vi "Write Input Action.vi"(8 "Error In":errorcluster, 10 "Input Action":T1, 11 "XBMC Ref":T2) -> (0 "Error Out":errorcluster, 3 "XBMC Ref":T2)   [LabVIEW 2013, in "LVH-XBMC.lvlib"]
uses:
  <vilib>/LabVIEW Hacker/XBMC/LVH-XBMC.lvlib
  <vilib>/LabVIEW Hacker/XBMC/Private/Type Defs/XBMC Ref.ctl
  <vilib>/httpClient/ClientHandle.ctl
  <vilib>/LabVIEW Hacker/XBMC/Private/Type Defs/Input.Action.ctl
  <vilib>/httpClient/LabVIEWHTTPClient.lvlib
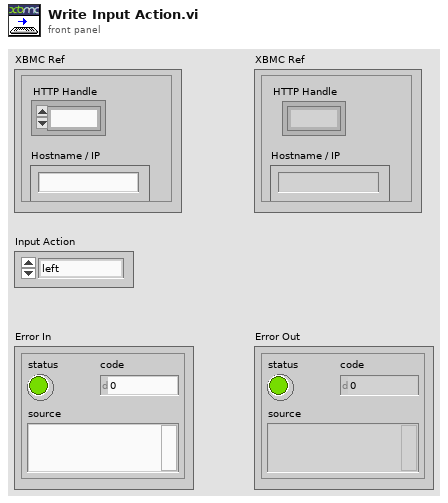
[diagram p1: front panel]
types:
  T1 = typedef "LVH-XBMC.lvlib/Input.Action.ctl" = enum16{"left", "right", "up", "down", "pageup", "pagedown", "select", "highlight", "parentdir", "parentfolder", "back", "previousmenu", "info", "pause", "stop", "skipnext", "skipprevious", "fullscreen", "aspectratio", "stepforward", "stepback", "bigstepforward", "bigstepback", "chapterorbigstepforward", "chapterorbigstepback", "osd", "showsubtitles", "nextsubtitle", "codecinfo", "nextpicture", "previouspicture", "zoomout", "zoomin", "playlist", "queue", "zoomnormal", "zoomlevel1", "zoomlevel2", "zoomlevel3", "zoomlevel4", "zoomlevel5", "zoomlevel6", "zoomlevel7", "zoomlevel8", "zoomlevel9", "nextcalibration", "resetcalibration", "analogmove", "rotate", "rotateccw", "close", "subtitledelayminus", "subtitledelay", "subtitledelayplus", "audiodelayminus", "audiodelay", "audiodelayplus", "subtitleshiftup", "subtitleshiftdown", "subtitlealign", "audionextlanguage", "verticalshiftup", "verticalshiftdown", "nextresolution", "audiotoggledigital", "number0", "number1", "number2", "number3", "number4", "number5", "number6", "number7", "number8", "number9", "osdleft", "osdright", "osdup", "osddown", "osdselect", "osdvalueplus", "osdvalueminus", "smallstepback", "fastforward", "rewind", "play", "playpause", "switchplayer", "delete", "copy", "move", "mplayerosd", "hidesubmenu", "screenshot", "rename", "togglewatched", "scanitem", "reloadkeymaps", "volumeup", "volumedown", "mute", "backspace", "scrollup", "scrolldown", "analogfastforward", "analogrewind", "moveitemup", "moveitemdown", "contextmenu", "shift", "symbols", "cursorleft", "cursorright", "showtime", "analogseekforward", "analogseekback", "showpreset", "presetlist", "nextpreset", "previouspreset", "lockpreset", "randompreset", "increasevisrating", "decreasevisrating", "showvideomenu", "enter", "increaserating", "decreaserating", "togglefullscreen", "nextscene", "previousscene", "nextletter", "prevletter", "jumpsms2", "jumpsms3", "jumpsms4", "jumpsms5", "jumpsms6", "jumpsms7", "jumpsms8", "jumpsms9", "filter", "filterclear", "filtersms2", "filtersms3", "filtersms4", "filtersms5", "filtersms6", "filtersms7", "filtersms8", "filtersms9", "firstpage", "lastpage", "guiprofile", "red", "green", "yellow", "blue", "increasepar", "decreasepar", "volampup", "volampdown", "createbookmark", "createepisodebookmark", "settingsreset", "settingslevelchange", "stereomode", "nextstereomode", "previousstereomode", "togglestereomode", "stereomodetomono", "channelup", "channeldown", "previouschannelgroup", "nextchannelgroup", "playpvr", "playpvrtv", "playpvrradio", "record", "leftclick", "rightclick", "middleclick", "doubleclick", "wheelup", "wheeldown", "mousedrag", "mousemove", "tap", "longpress", "pangesture", "zoomgesture", "rotategesture", "swipeleft", "swiperight", "swipeup", "swipedown", "noop"}
  T2 = typedef "LVH-XBMC.lvlib/XBMC Ref.ctl" = cluster{"HTTP Handle":T3, "Hostname / IP":string}
  T3 = typedef "LabVIEWHTTPClient.lvlib/ClientHandle.ctl" = refnum<k1>
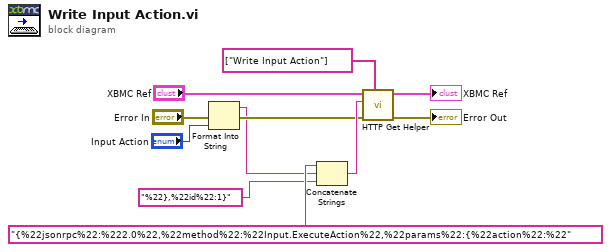
[diagram p0: block diagram]
diagram:
  n1 = Format Into String(error in="Error In", "Input Action") -> (resulting string=w1:string, error out=w2:errorcluster)  [unwired: 2 in]
  n2 = Concatenate Strings("{%22jsonrpc%22:%222.0%22,%22method%22:%22Input.ExecuteAction%22,%22params%22:{%22action%22:%22" ("string"), w1, "%22},%22id%22:1}" ("string")) -> (w8:string)
  n3 = call <vilib>:"HTTP Get Helper.vi"("Error Arguments"=string[] ["Write Input Action"], "Error In"=w2, "JSON Request"=w8, "XBMC Ref"="XBMC Ref") -> ("Error Out"=→"Error Out":errorcluster, "XBMC Ref"=→"XBMC Ref":T2)  [unwired: 6 in]
